vi "multi_publisher.vi"() -> ()   [LabVIEW 2014]
panel:
  out "JSON字符串 4":string
  out "JSON字符串 3":string
  in  "停止 2":bool
  in  "停止":bool
  out "JSON字符串 2":string
  out "JSON字符串":string
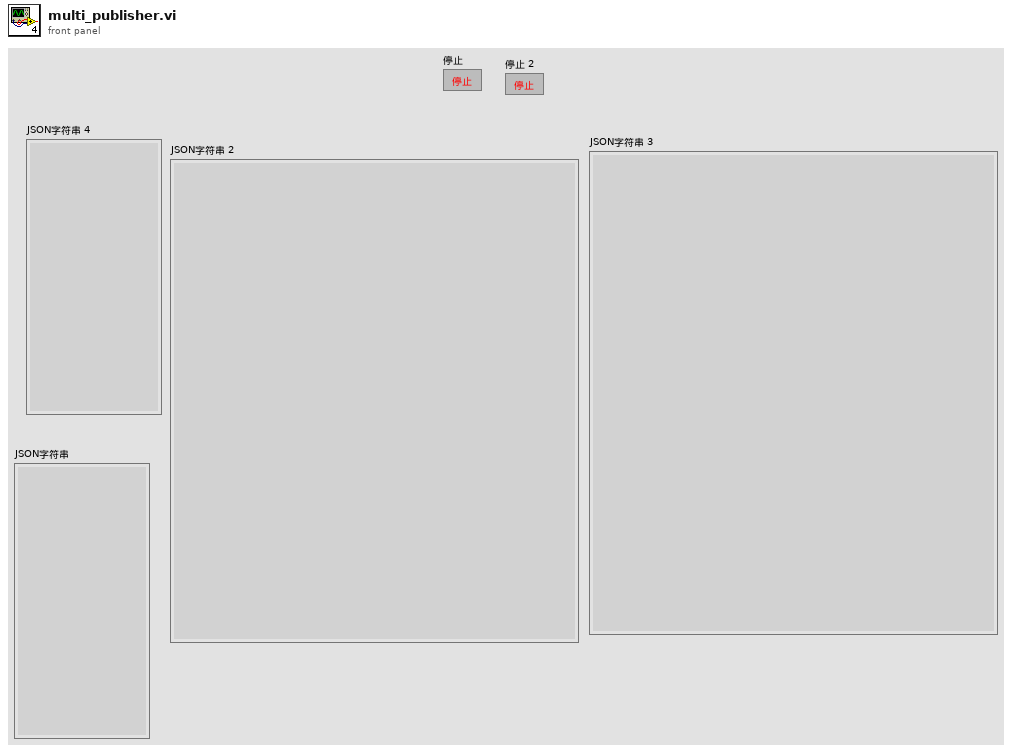
[diagram p1: front panel]
types:
  T1 = cluster{"op":string, "topic":string, "type":string}
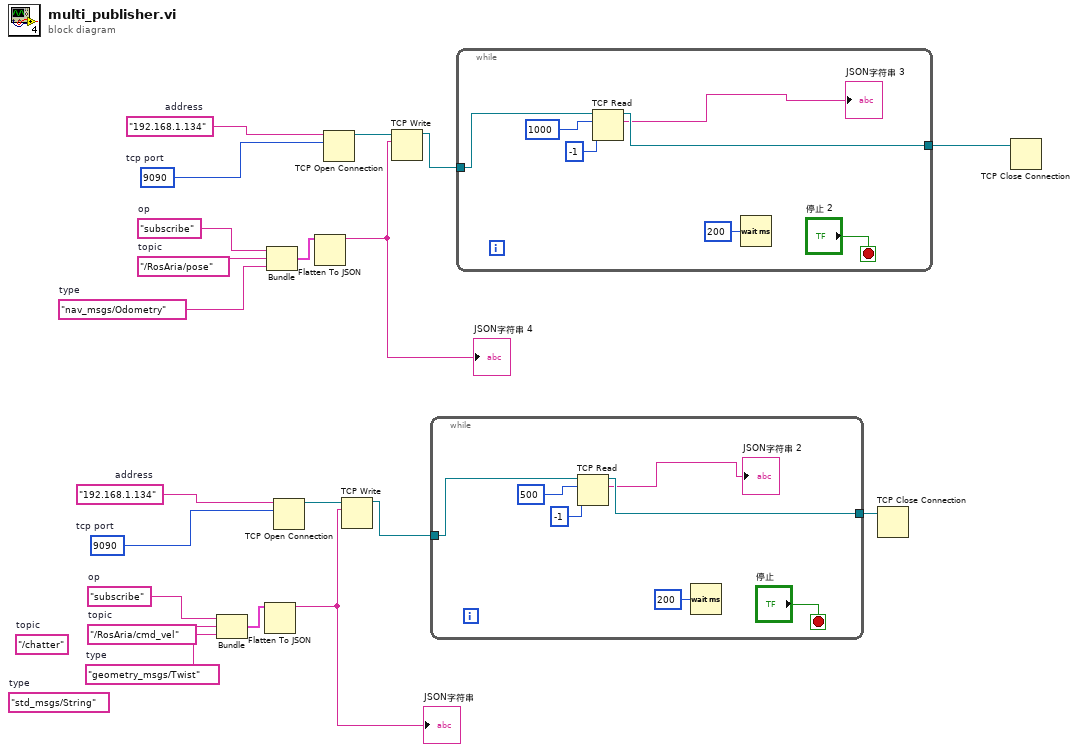
[diagram p0: block diagram]
diagram:
  w7 = "nav_msgs/Odometry"  # type
  w9 = "subscribe"  # op
  w8 = "/RosAria/pose"  # topic
  w2 = u16 9090  # tcp port
  w1 = "192.168.1.134"  # address
  (unwired) "std_msgs/String"  # type
  (unwired) "/chatter"  # topic
  w14 = "geometry_msgs/Twist"  # type
  w12 = "subscribe"  # op
  w13 = "/RosAria/cmd_vel"  # topic
  w19 = u16 9090  # tcp port
  w20 = "192.168.1.134"  # address
  n1 = Bundle("op"=w12, "topic"=w13, "type"=w14) -> (w15:T1)  [unwired: 1 in]
  n2 = Flatten To JSON(anything=w15) -> (JSON string=w11:string)  [unwired: 2 in, 1 out]
  "JSON字符串" <- w11
  n3 = Bundle("op"=w9, "topic"=w8, "type"=w7) -> (w6:T1)  [unwired: 1 in]
  n4 = TCP Open Connection(address=w20, remote port or service name=w19) -> (connection ID=w17:refnum<k5>)  [unwired: 3 in, 1 out]
  n5 = Flatten To JSON(anything=w6) -> (JSON string=w10:string)  [unwired: 2 in, 1 out]
  "JSON字符串 4" <- w10
  n6 = TCP Open Connection(address=w1, remote port or service name=w2) -> (connection ID=w4:refnum<k5>)  [unwired: 3 in, 1 out]
  n7 = TCP Write(connection ID=w17, data in=w11) -> (connection ID out=w16:refnum<k5>)  [unwired: 2 in, 2 out]
  n8 = TCP Write(connection ID=w4, data in=w10) -> (connection ID out=w5:refnum<k5>)  [unwired: 2 in, 2 out]
  n9 = while {
    tunnel: [w25] -> w18
    tunnel: w16 -> [w26]
    stop <- "停止" stop-if-true
    n10 = TCP Read(connection ID=w26, bytes to read=500 ("读取的字节"), 9:-1 ("超时毫秒(25000)")) -> (connection ID out=w25:refnum<k5>, data out=→"JSON字符串 2":string)  [unwired: 2 in, 1 out]
    n11 = Wait (ms)(milliseconds to wait=u32 200 ("等待时间（毫秒）")) -> ()  [unwired: 1 out]
  }
  n12 = while {
    tunnel: [w32] -> w3
    tunnel: w5 -> [w33]
    stop <- "停止 2" stop-if-true
    n13 = TCP Read(connection ID=w33, bytes to read=1000 ("读取的字节"), 9:-1 ("超时毫秒(25000)")) -> (connection ID out=w32:refnum<k5>, data out=→"JSON字符串 3":string)  [unwired: 2 in, 1 out]
    n14 = Wait (ms)(milliseconds to wait=u32 200 ("等待时间（毫秒）")) -> ()  [unwired: 1 out]
  }
  n15 = TCP Close Connection(connection ID=w18) -> ()  [unwired: 2 in, 2 out]
  n16 = TCP Close Connection(connection ID=w3) -> ()  [unwired: 2 in, 2 out]
